vi "Vision Research Phantom Series PhCon PhGetAllIpCameras.vi"(5 "Error In (no error)":errorcluster) -> (14 "pCnt [out]":u32, 15 "pCam [out]":u8[](array[numeric]), 19 "Error Out":errorcluster)   [LabVIEW 2013, in "VRI.lvlib"]
doc: "PhGetAllIpCameras\nHRESULT PhGetAllIpCameras(PUINT pCnt, PCAMERAID pCam)\n\nParameters\npCnt [out]\n Address where the discovered camera count will be stored.\npCam [out]\n Buffer to be filled with CAMERAID elements describing discovered cameras.\n\nReturn Value\nThe function returns ERR_Ok in case of success or an error code, otherwise. To get extended error information call PhGetErrorMessage.\n\nRemarks\nIt provides a quick option for getting information about connected cameras. It does not affect or interact with current camera pool.\n\nRequired Header\nPhCon.h"
uses:
  VRI.lvlib
  Phantom DLLs/PhCon.Dll
panel:
  # "For instructions on the use of this VI, press Ctrl+H to display the help window and move the mouse over the icon, controls, and indicators"
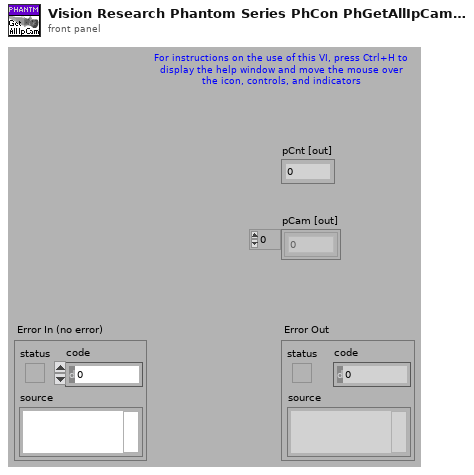
[diagram p1: front panel]
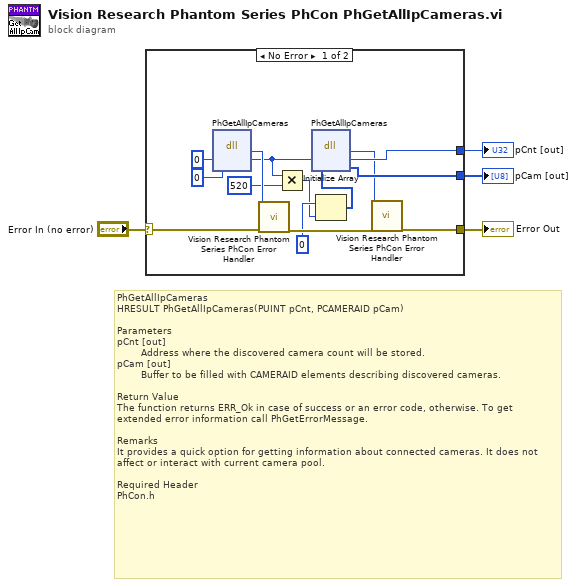
[diagram p0: block diagram]
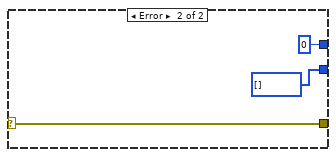
[diagram p2: hidden frame]
diagram:
  # "PhGetAllIpCameras\nHRESULT PhGetAllIpCameras(PUINT pCnt, PCAMERAID pCam)\n\nParameters\npCnt [out]\n\t       Address where the discovered camera count will be stored.\npCam [out]\n        Buffer to be filled with CAMERAID elements describing discovered cameras.\n\nReturn Value\nThe function returns ERR_Ok in case of success or an error code, otherwise. To get extended error information call PhGetErrorMessage.\n\nRemarks\nIt provides a quick option for getting information about connected cameras. It does not affect or interact with current camera pool.\n\nRequired Header\nPhCon.h"
  n1 = case shown="No Error" "Error In (no error)" {
    selector: "Error In (no error)" -> [w18 w21]
    tunnel: [w17 w21] -> w3
    tunnel: [w16 u8[] [] ("pCam")] -> w1
    tunnel: [w15 u32 0 ("pCnt")] -> w2
    frame No Error {
      n2 = dll-call lib="C:/Projects/SDK/64-bit/Vision Research Phantom Series Labview Driver/Phantom DLLs/PhCon.dll" fn="PhGetAllIpCameras"("pCnt"=u32 0, "pCam"=0) -> ("HRESULT"=w10:i32, "pCnt"=w8:u32)  [unwired: 3 in, 3 out]
      n3 = call "Vision Research Phantom Series PhCon Error Handler.vi"("ErrNo"=w10, "Error In (no error)"=w18) -> ("Error Out"=w11:errorcluster)  [unwired: 17 out]
      n4 = Multiply(x=w8, y=u32 520) -> (x*y=w6:u32)
      n5 = Initialize Array(u8 0 ("pCam"), w6) -> (w5:u8[])
      n6 = dll-call lib="C:/Projects/SDK/64-bit/Vision Research Phantom Series Labview Driver/Phantom DLLs/PhCon.dll" fn="PhGetAllIpCameras"("pCnt"=w8, "pCam"=w5) -> ("HRESULT"=w14:i32, "pCnt"=w15:u32, "pCam"=w16:u8[])  [unwired: 3 in, 2 out]
      n7 = call "Vision Research Phantom Series PhCon Error Handler.vi"("ErrNo"=w14, "Error In (no error)"=w11) -> ("Error Out"=w17:errorcluster)  [unwired: 17 out]
    }
    frame Error {
    }
  }
  "Error Out" <- w3
  "pCnt [out]" <- w2
  "pCam [out]" <- w1
